vi "BundleData.vi"(11 "DataIn":dbl[][](array[numeric])) -> (3 "DataOut":cluster{"数组":dbl[]}[](array[cluster]))   [LabVIEW 2018, in "DataDisplay.lvlib"]
uses:
  DataDisplay.lvlib
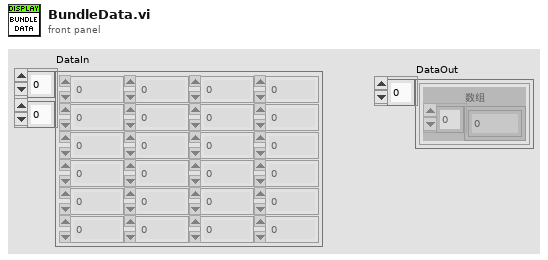
[diagram p1: front panel]
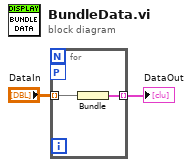
[diagram p0: block diagram]
diagram:
  n1 = for {
    tunnel: "DataIn" -> [w4] mode=indexing
    tunnel: [w3] -> w1 mode=indexing
    workers-P: _ -> [_]
    n2 = Bundle("DataIn"=w4) -> (w3:cluster{"DataIn":dbl[]})  [unwired: 1 in]
  }
  "DataOut" <- w1
